vi "获取环境参数 (子VI).vi"   [LabVIEW 2016, in "数据传输系统.lvlib"]
types:
  T1 = enum16{"CODMn", "PH", "氨氮", "总氮", "总磷", "CODCr", "电导率", "水温", "DO", "浊度", "叶绿素", "藻密度"}
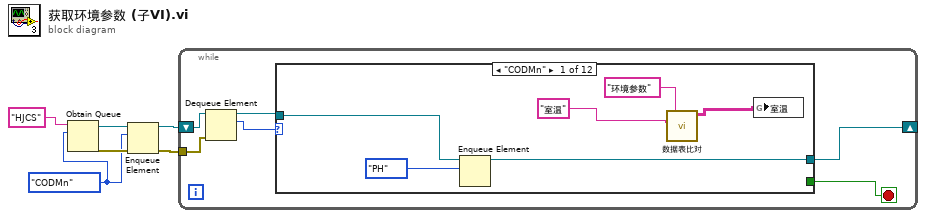
[diagram p0: block diagram]
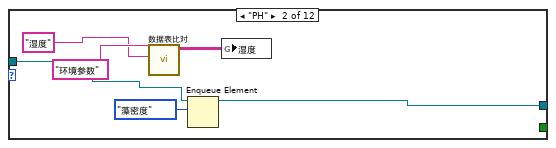
[diagram p2: hidden frame]
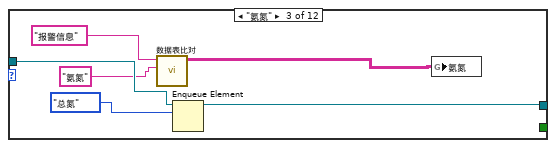
[diagram p3: hidden frame]
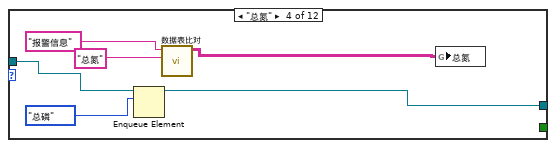
[diagram p4: hidden frame]
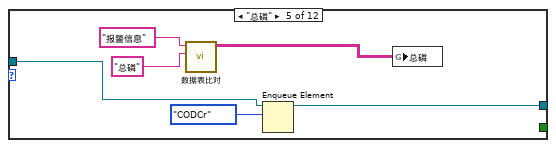
[diagram p5: hidden frame]
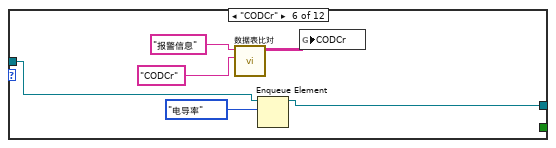
[diagram p6: hidden frame]
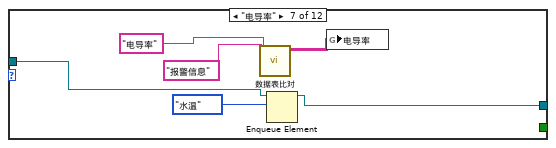
[diagram p7: hidden frame]
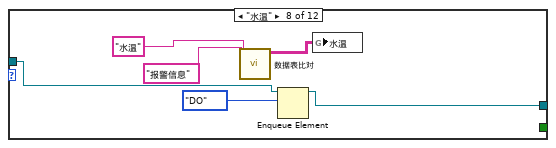
[diagram p8: hidden frame]
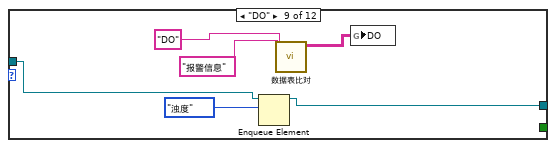
[diagram p9: hidden frame]
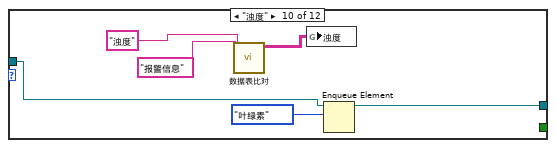
[diagram p10: hidden frame]
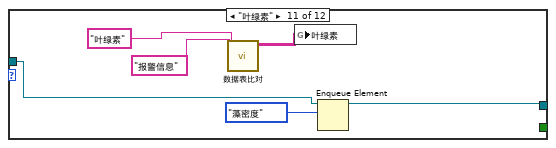
[diagram p11: hidden frame]
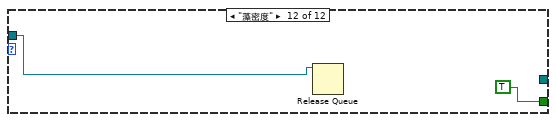
[diagram p12: hidden frame]
diagram:
  w1 = T1."CODMn"
  n1 = Obtain Queue(name (unnamed)="HJCS" ("名称（未命名）"), element data type=w1) -> (queue out=w5:refnum<queue>, error out=w2:errorcluster)  [unwired: 3 in, 1 out]
  n2 = Enqueue Element(queue=w5, element=w1, error in (no error)=w2) -> (queue out=w4:refnum<queue>, error out=w3:errorcluster)  [unwired: 1 in, 1 out]
  n3 = while {
    shift-right: [w10] -> _
    shift-left: w4 -> [w12]
    tunnel: w3 -> [w9]
    stop <- w7 stop-if-true
    n4 = Dequeue Element(queue=w12, error in (no error)=w9) -> (queue out=w11:refnum<queue>, element=w8:T1)  [unwired: 1 in, 2 out]
    n5 = case shown="\"CODMn\"" w8 {
      tunnel: w11 -> [w18 w24 w29 w36 w41 w46 w50 w56 w62 w68 w74 w80]
      tunnel: [w17 w23 w30 w35 w40 w45 w49 w55 w61 w67 w73 _] -> w10
      tunnel: [_ _ _ _ _ _ _ _ _ _ _ TRUE] -> w7
      frame "CODMn" {
        n6 = Enqueue Element(queue=w18, element=T1."PH") -> (queue out=w17:refnum<queue>)  [unwired: 2 in, 2 out]
        n7 = call "数据表比对.vi"("仪器日志参数"="室温" ("元素"), "table输入"="环境参数" ("新元素/子数组")) -> ("待发送数据"=w14:string[][])  [unwired: 7 in, 2 out]
        n8 = global write "全局 环境参数.vi" "室温"(w14) -> ()
      }
      frame "PH" {
        n9 = call "数据表比对.vi"("仪器日志参数"="湿度" ("元素"), "table输入"="环境参数" ("新元素/子数组")) -> ("待发送数据"=w20:string[][])  [unwired: 7 in, 2 out]
        n10 = Enqueue Element(queue=w24, element=T1."藻密度") -> (queue out=w23:refnum<queue>)  [unwired: 2 in, 2 out]
        n11 = global write "全局 环境参数.vi" "湿度"(w20) -> ()
      }
      frame "氨氮" {
        n12 = call "数据表比对.vi"("仪器日志参数"="氨氮" ("元素"), "table输入"="报警信息" ("新元素/子数组")) -> ("待发送数据"=w27:string[][])  [unwired: 7 in, 2 out]
        n13 = Enqueue Element(queue=w29, element=T1."总氮") -> (queue out=w30:refnum<queue>)  [unwired: 2 in, 2 out]
        n14 = global write "全局 所有参数.vi" "氨氮"(w27) -> ()
      }
      frame "总氮" {
        n15 = Enqueue Element(queue=w36, element=T1."总磷") -> (queue out=w35:refnum<queue>)  [unwired: 2 in, 2 out]
        n16 = call "数据表比对.vi"("仪器日志参数"="总氮" ("元素"), "table输入"="报警信息" ("新元素/子数组")) -> ("待发送数据"=w33:string[][])  [unwired: 7 in, 2 out]
        n17 = global write "全局 所有参数.vi" "总氮"(w33) -> ()
      }
      frame "总磷" {
        n18 = call "数据表比对.vi"("仪器日志参数"="总磷" ("元素"), "table输入"="报警信息" ("新元素/子数组")) -> ("待发送数据"=w39:string[][])  [unwired: 7 in, 2 out]
        n19 = Enqueue Element(queue=w41, element=T1."CODCr") -> (queue out=w40:refnum<queue>)  [unwired: 2 in, 2 out]
        n20 = global write "全局 所有参数.vi" "总磷"(w39) -> ()
      }
      frame "CODCr" {
        n21 = call "数据表比对.vi"("仪器日志参数"="CODCr" ("元素"), "table输入"="报警信息" ("新元素/子数组")) -> ("待发送数据"=w48:string[][])  [unwired: 7 in, 2 out]
        n22 = Enqueue Element(queue=w46, element=T1."电导率") -> (queue out=w45:refnum<queue>)  [unwired: 2 in, 2 out]
        n23 = global write "全局 所有参数.vi" "CODCr"(w48) -> ()
      }
      frame "电导率" {
        n24 = call "数据表比对.vi"("查询元素输入"="电导率" ("元素"), "table输入"="报警信息" ("新元素/子数组")) -> ("待发送数据"=w52:string[][])  [unwired: 7 in, 2 out]
        n25 = Enqueue Element(queue=w50, element=T1."水温") -> (queue out=w49:refnum<queue>)  [unwired: 2 in, 2 out]
        n26 = global write "全局 所有参数.vi" "电导率"(w52) -> ()
      }
      frame "水温" {
        n27 = call "数据表比对.vi"("查询元素输入"="水温" ("元素"), "table输入"="报警信息" ("新元素/子数组")) -> ("待发送数据"=w58:string[][])  [unwired: 7 in, 2 out]
        n28 = Enqueue Element(queue=w56, element=T1."DO") -> (queue out=w55:refnum<queue>)  [unwired: 2 in, 2 out]
        n29 = global write "全局 所有参数.vi" "水温"(w58) -> ()
      }
      frame "DO" {
        n30 = Enqueue Element(queue=w62, element=T1."浊度") -> (queue out=w61:refnum<queue>)  [unwired: 2 in, 2 out]
        n31 = call "数据表比对.vi"("查询元素输入"="DO" ("元素"), "table输入"="报警信息" ("新元素/子数组")) -> ("待发送数据"=w64:string[][])  [unwired: 7 in, 2 out]
        n32 = global write "全局 所有参数.vi" "DO"(w64) -> ()
      }
      frame "浊度" {
        n33 = call "数据表比对.vi"("查询元素输入"="浊度" ("元素"), "table输入"="报警信息" ("新元素/子数组")) -> ("待发送数据"=w69:string[][])  [unwired: 7 in, 2 out]
        n34 = global write "全局 所有参数.vi" "浊度"(w69) -> ()
        n35 = Enqueue Element(queue=w68, element=T1."叶绿素") -> (queue out=w67:refnum<queue>)  [unwired: 2 in, 2 out]
      }
      frame "叶绿素" {
        n36 = call "数据表比对.vi"("查询元素输入"="叶绿素" ("元素"), "table输入"="报警信息" ("新元素/子数组")) -> ("待发送数据"=w75:string[][])  [unwired: 7 in, 2 out]
        n37 = global write "全局 所有参数.vi" "叶绿素"(w75) -> ()
        n38 = Enqueue Element(queue=w74, element=T1."藻密度") -> (queue out=w73:refnum<queue>)  [unwired: 2 in, 2 out]
      }
      frame "藻密度" {
        n39 = Release Queue(queue=w80) -> ()  [unwired: 2 in, 3 out]
      }
    }
  }
